vi "CTRE_Phoenix_CANifier_GetCustomParameter.vi"(6 "timeoutMs":i32, 8 "error in":errorcluster, 10 "paramIndex":i32, 11 "CTRE_CANifier_DeviceRef":T1) -> (0 "error out":errorcluster, 2 "readValue":i32, 3 "CTRE_CANifier_DeviceRef":T1)   [LabVIEW 2017]
doc: "Returns the selected custom parameter value."
uses:
  CTRE_CANifier_DeviceRef.ctl
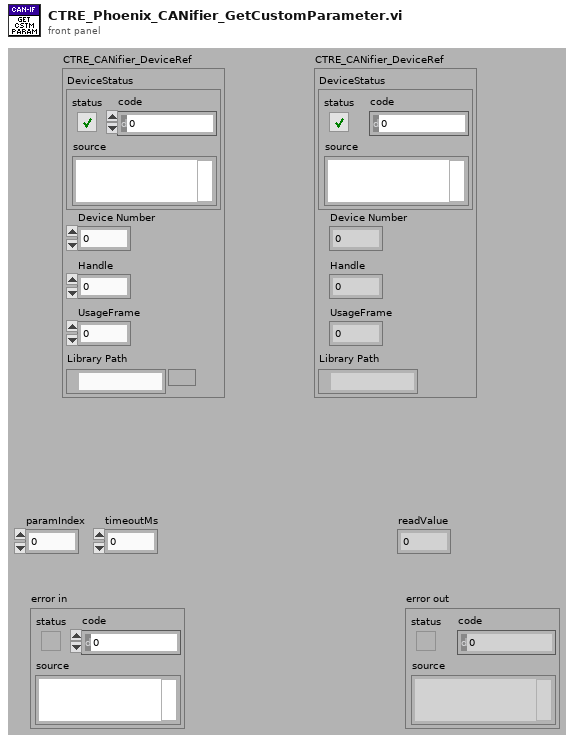
[diagram p1: front panel]
types:
  T1 = typedef "CTRE_CANifier_DeviceRef.ctl" = cluster{"DeviceStatus":errorcluster, "Device Number":u8, "Handle":u64, "UsageFrame":u32, "Library Path":path}
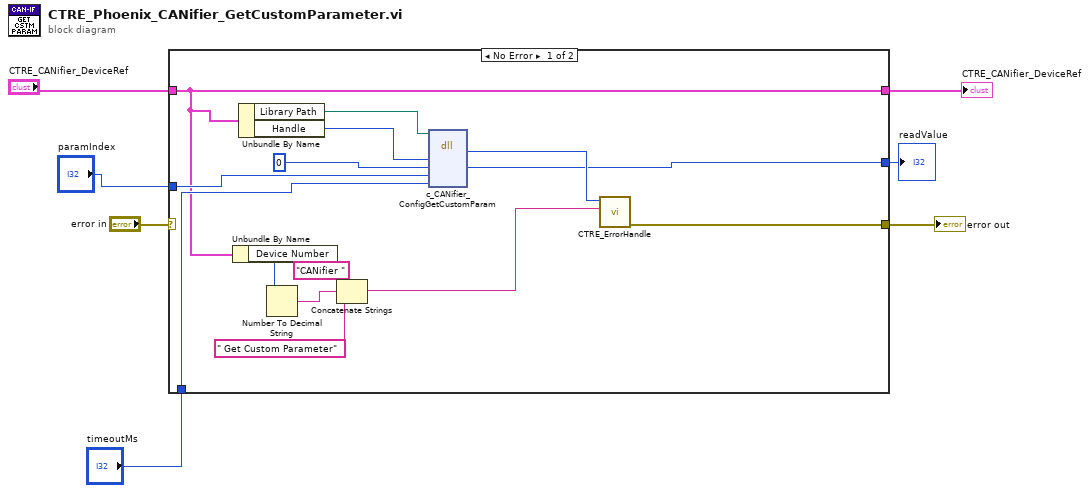
[diagram p0: block diagram]
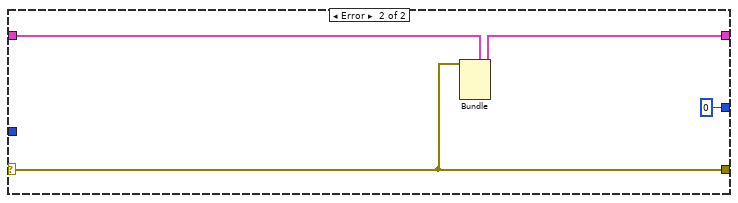
[diagram p2: hidden frame]
diagram:
  n1 = case shown="No Error" "error in" {
    selector: "error in" -> [_ w24]
    tunnel: "CTRE_CANifier_DeviceRef" -> [w10 w25]
    tunnel: [w21 w24] -> w7
    tunnel: [w10 w23] -> w1
    tunnel: "paramIndex" -> [w13 _]
    tunnel: "timeoutMs" -> [w12 _]
    tunnel: [w11 0 ("readValue")] -> w3
    frame No Error {
      n2 = Unbundle By Name(w10) -> ("Device Number"=w17:u8)
      n3 = Unbundle By Name(w10) -> ("Library Path"=w9:path, "Handle"=w8:u64)
      n4 = Number To Decimal String(number=w17) -> (decimal integer string=w19:string)  [unwired: 1 in]
      n5 = Concatenate Strings("CANifier " ("string"), w19, " Get Custom Parameter" ("string")) -> (w15:string)
      n6 = dll-call lib="?" fn="c_CANifier_ConfigGetCustomParam"(path in=w9, "handle"=w8, "readValue"=0, "paramIndex"=w13, "timeoutMs"=w12) -> ("return type"=w16:i32, "readValue"=w11:i32)  [unwired: 5 in, 2 out]
      n7 = call "CTRE_ErrorHandle.vi"("origin"=w15, "code"=w16) -> ("error out"=w21:errorcluster)  [unwired: 9 in]
    }
    frame Error {
      n8 = Bundle(cluster=w25, "DeviceStatus"=w24) -> (w23:T1)  [unwired: 4 in]
    }
  }
  "error out" <- w7
  "readValue" <- w3
  "CTRE_CANifier_DeviceRef" <- w1
